vi "Log Message.vi"(8 "error in (no error)":errorcluster, 10 "Logging Level":T1, 11 "Message":string) -> (0 "error out":errorcluster)   [LabVIEW 2019, in "Logger.lvlib" / "Logger.lvclass"]
uses:
  Logger.lvclass
  Type Defs/Logging Level.ctl
  Type Defs/Logging Message.ctl
  Global Variables/Logging Configuration.vi
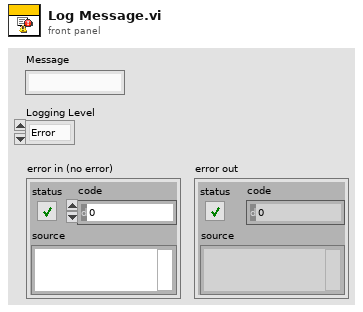
[diagram p1: front panel]
types:
  T1 = typedef "Logger.lvlib/Logger.lvclass/Logging Level.ctl" = enum16{"Error", "Warning", "Info", "Trace"}
  T2 = typedef "Logger.lvlib/Logger.lvclass/Logging Message.ctl" = cluster{"Time Stamp":timestamp, "Logging Level":T1, "VI Name":string, "Message":string}
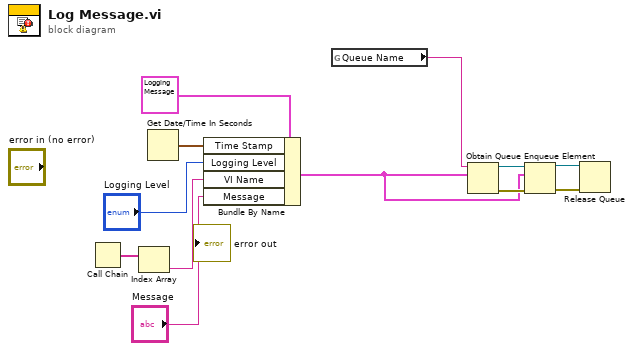
[diagram p0: block diagram]
diagram:
  n1 = Call Chain() -> (call chain=w10:string[])
  n2 = Index Array(array=w10) -> (element=w9:string)  [unwired: 1 in]
  n3 = Get Date/Time In Seconds() -> (seconds since 1Jan1904=w7:timestamp)
  n4 = Bundle By Name(cluster=T2 {"Time Stamp"=timestamp(0 s since 1904-01-01), "Logging Level"=enum."Error", "VI Name"="", "Message"=""} ("Logging Message"), "Time Stamp"=w7, "Logging Level"="Logging Level", "VI Name"=w9, "Message"="Message") -> (w3:T2)
  n5 = global read "Logging Configuration.vi" "Queue Name"() -> (w4:string)
  n6 = Obtain Queue(name (unnamed)=w4, element data type=w3) -> (queue out=w6:refnum<queue>, error out=w5:errorcluster)  [unwired: 3 in, 1 out]
  n7 = Enqueue Element(queue=w6, element=w3, error in (no error)=w5) -> (queue out=w2:refnum<queue>, error out=w1:errorcluster)  [unwired: 1 in, 1 out]
  n8 = Release Queue(queue=w2, error in (no error)=w1) -> ()  [unwired: 1 in, 3 out]
